vi "Post (U16).vi"(6 "timestamp in":timestamp, 7 "PV name":string, 8 "error in (no error)":errorcluster, 10 "value in":u16, 11 "Server in":refnum<class "Server.lvclass">) -> (0 "error out":errorcluster, 2 "value out":u16, 3 "Server out":refnum<class "Server.lvclass">, 4 "timestamp out":timestamp)   [LabVIEW 2020, in "PV Access.lvlib" / "PVA Server.lvlib" / "Server.lvclass"]
uses:
  Server.lvclass
  Server.lvclass/Server.ctl
  25a0afa2-78cc-4e41-9cb9-729b0faefda4.vi
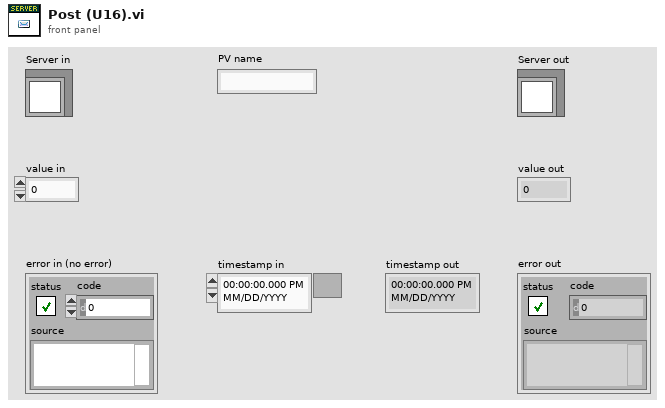
[diagram p1: front panel]
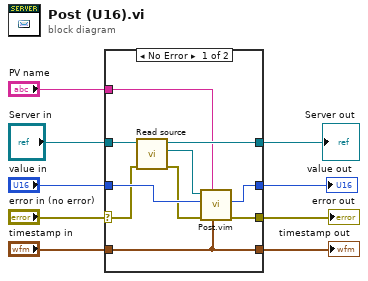
[diagram p0: block diagram]
diagram:
  n1 = case shown="No Error" "error in (no error)" {
    selector: "error in (no error)" -> [w12 w23]
    tunnel: [w13 w23] -> w3
    tunnel: [w18 w22] -> w1
    tunnel: "Server in" -> [w19 w22]
    tunnel: "PV name" -> [w14 _]
    tunnel: "value in" -> [w16 w21]
    tunnel: [w17 w21] -> w4
    tunnel: "timestamp in" -> [w10 w20]
    tunnel: [w10 w20] -> w2
    frame No Error {
      n2 = call "Read source.vi"("error in (no error)"=w12, "Server in"=w19) -> ("error out"=w11:errorcluster, "Source"=w15:refnum<class "Source.lvclass">, "Server out"=w18:refnum<class "Server.lvclass">)  [unwired: 7 in]
      n3 = call "Post.vim"("timestamp in"=w10, "PV name"=w14, "error in"=w11, "value in"=w16, "Source in"=w15) -> ("error out"=w13:errorcluster, "value out"=w17:u16)  [unwired: 3 in, 2 out]
    }
    frame Error {
    }
  }
  "error out" <- w3
  "Server out" <- w1
  "value out" <- w4
  "timestamp out" <- w2
